vi "Remove Outliers (single).vi"(8 "error in (no error)":errorcluster, 9 "Y Lower":dbl, 10 "Y Upper":dbl, 11 "XY-data":cluster{"X-array":dbl[], "Y-array":dbl[]}) -> (0 "error out":errorcluster, 3 "XY-data out":cluster{"X-array":dbl[], "Y-array":dbl[]} {"Y-array" format="%.2p"; "X-array" format="%.2p"})   [LabVIEW 2016, in "xy_utilities.lvlib"]
doc: "Remove outliers from the y array of <b>XY-data</b> between <b>Y Upper</b> and <b>Y Lower</b> limits.\n\nWire data to the data input to determine the polymorphic instance to use or manually select the instance."
uses:
  xy_utilities.lvlib
  <vilib>/Analysis/6fits.llb/Remove Outliers (Range).vi
  <vilib>/Analysis/NI_AALPro.lvlib
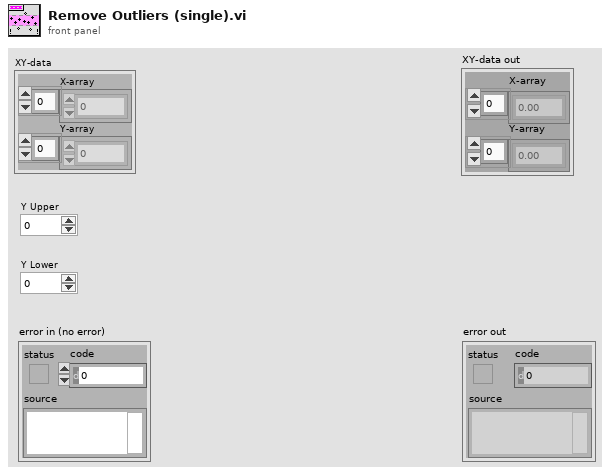
[diagram p1: front panel]
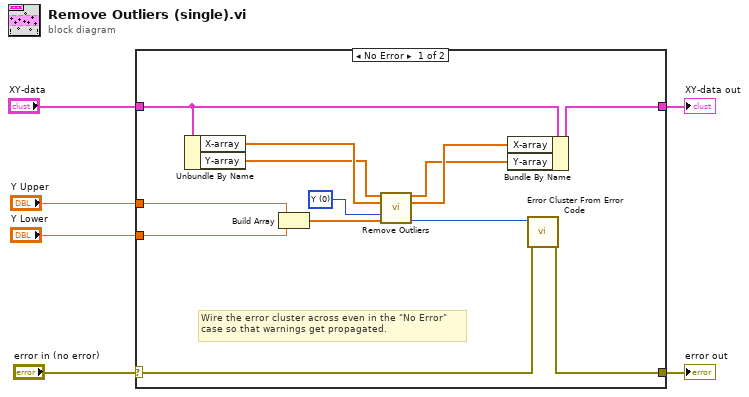
[diagram p0: block diagram]
diagram:
  n1 = case shown="No Error" "error in (no error)" {
    selector: "error in (no error)" -> [w9 w21]
    tunnel: [w8 w21] -> w5
    tunnel: "XY-data" -> [w19 w20]
    tunnel: [w18 w20] -> w3
    tunnel: "Y Lower" -> [w16 _]
    tunnel: "Y Upper" -> [w17 _]
    frame No Error {
      w7 = u16 0 items=["Y", "X", "X and Y"] ("range type")
      # "Wire the error cluster across even in the \"No Error\"\ncase so that warnings get propagated."
      n2 = Unbundle By Name(w19) -> ("X-array"=w14:dbl[], "Y-array"=w11:dbl[])
      n3 = Build Array(w17, w16) -> (w15:dbl[])
      n4 = call-poly <vilib>:"Remove Outliers.vi"("Y"=w11, "X"=w14, "range type"=w7, "Range"=w15) -> ("Y Out"=w12:dbl[], "X Out"=w13:dbl[], "error"=w10:i32)  [unwired: 7 in, 2 out]
      n5 = Bundle By Name(cluster=w19, "X-array"=w13, "Y-array"=w12) -> (w18:cluster{"X-array":dbl[], "Y-array":dbl[]})
      n6 = call <vilib>:"Error Cluster From Error Code.vi"("error in (no error)"=w9, "error code (0)"=w10) -> ("error out"=w8:errorcluster)  [unwired: 7 in]
    }
    frame Error {
    }
  }
  "error out" <- w5
  "XY-data out" <- w3
